vi "[PC]UpdateGlobVar.vi"   [LabVIEW 2018]
uses:
  TypeDef/ControllerState.ctl
  RT/[GlobVar]SensorState.vi
types:
  T1 = typedef "ControllerState.ctl" = enum16{"Idle", "Vorheizen", "Brühen", "Emergency-Stop"}
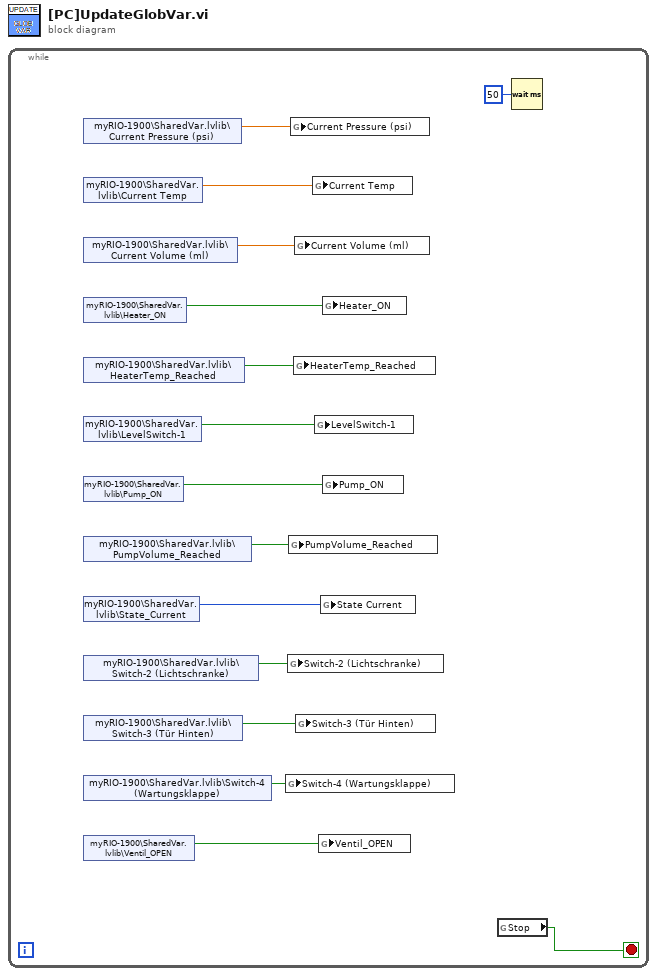
[diagram p0: block diagram]
diagram:
  n1 = while {
    stop <- w2 stop-if-true
    n2 = shared-variable "myRIO-1900\\SharedVar.lvlib\\Current Pressure (psi)"() -> (w3:dbl)  [unwired: 1 in, 1 out]
    n3 = shared-variable "myRIO-1900\\SharedVar.lvlib\\Current Temp"() -> (w4:dbl)  [unwired: 1 in, 1 out]
    n4 = shared-variable "myRIO-1900\\SharedVar.lvlib\\Current Volume (ml)"() -> (w5:dbl)  [unwired: 1 in, 1 out]
    n5 = shared-variable "myRIO-1900\\SharedVar.lvlib\\Heater_ON"() -> (w6:bool)  [unwired: 1 in, 1 out]
    n6 = shared-variable "myRIO-1900\\SharedVar.lvlib\\HeaterTemp_Reached"() -> (w7:bool)  [unwired: 1 in, 1 out]
    n7 = shared-variable "myRIO-1900\\SharedVar.lvlib\\LevelSwitch-1"() -> (w8:bool)  [unwired: 1 in, 1 out]
    n8 = shared-variable "myRIO-1900\\SharedVar.lvlib\\Pump_ON"() -> (w9:bool)  [unwired: 1 in, 1 out]
    n9 = shared-variable "myRIO-1900\\SharedVar.lvlib\\PumpVolume_Reached"() -> (w10:bool)  [unwired: 1 in, 1 out]
    n10 = shared-variable "myRIO-1900\\SharedVar.lvlib\\State_Current"() -> (w11:T1)  [unwired: 1 in, 1 out]
    n11 = shared-variable "myRIO-1900\\SharedVar.lvlib\\Switch-2 (Lichtschranke)"() -> (w12:bool)  [unwired: 1 in, 1 out]
    n12 = shared-variable "myRIO-1900\\SharedVar.lvlib\\Switch-3 (Tür Hinten)"() -> (w13:bool)  [unwired: 1 in, 1 out]
    n13 = shared-variable "myRIO-1900\\SharedVar.lvlib\\Switch-4 (Wartungsklappe)"() -> (w14:bool)  [unwired: 1 in, 1 out]
    n14 = shared-variable "myRIO-1900\\SharedVar.lvlib\\Ventil_OPEN"() -> (w15:bool)  [unwired: 1 in, 1 out]
    n15 = global write "[GlobVar]SensorState.vi" "Switch-4 (Wartungsklappe)"(w14) -> ()
    n16 = global write "[GlobVar]SensorState.vi" "Switch-2 (Lichtschranke)"(w12) -> ()
    n17 = global write "[GlobVar]SensorState.vi" "PumpVolume_Reached"(w10) -> ()
    n18 = global write "[GlobVar]SensorState.vi" "Current Pressure (psi)"(w3) -> ()
    n19 = global write "[GlobVar]SensorState.vi" "HeaterTemp_Reached"(w7) -> ()
    n20 = global write "[GlobVar]SensorState.vi" "Current Volume (ml)"(w5) -> ()
    n21 = global write "[GlobVar]SensorState.vi" "Switch-3 (Tür Hinten)"(w13) -> ()
    n22 = global write "[GlobVar]SensorState.vi" "Current Temp"(w4) -> ()
    n23 = global write "[GlobVar]SensorState.vi" "LevelSwitch-1"(w8) -> ()
    n24 = global write "[GlobVar]SensorState.vi" "Ventil_OPEN"(w15) -> ()
    n25 = global write "[GlobVar]SensorState.vi" "State Current"(w11) -> ()
    n26 = global write "[GlobVar]SensorState.vi" "Heater_ON"(w6) -> ()
    n27 = global write "[GlobVar]SensorState.vi" "Pump_ON"(w9) -> ()
    n28 = global read "[GlobVar]SensorState.vi" "Stop"() -> (w2:bool)
    n29 = Wait (ms)(milliseconds to wait=u32 50) -> ()  [unwired: 1 out]
  }
